vi "init.vi"(6 "Space size":i32=100000, 7 "Cleaneup":bool, 8 "error in (no error)":errorcluster) -> (0 "error out":errorcluster)   [LabVIEW 2015]
doc: "Initialize the tuple space naming it Spacename and reserving Space size locations for tuple. \nIf Cleanup is set to TRUE the pace will be initialized even if containing data.\nUse Cleneup=TRUE Spacesize=0 to deallocate all memory."
uses:
  LI_states.ctl
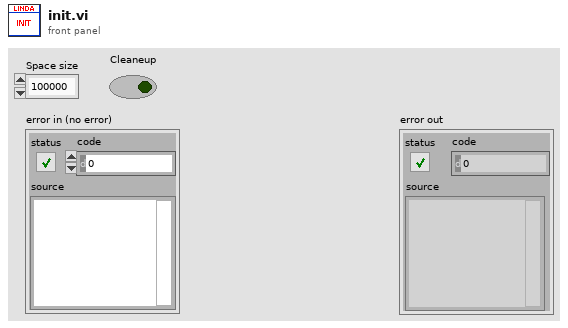
[diagram p1: front panel]
types:
  T1 = typedef "LI_states.ctl" = enum16{"Out", "In", "Rd", "Inp", "Rdp", "Init", "Cleanup", "RdAll"}
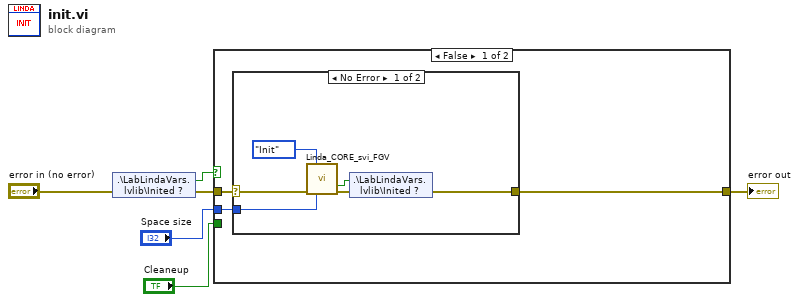
[diagram p0: block diagram]
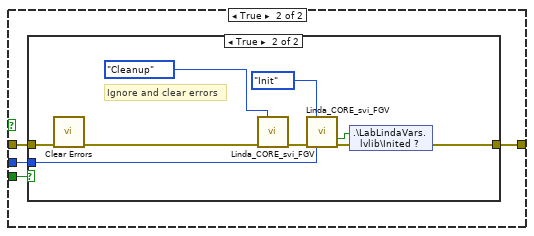
[diagram p3: hidden frame]
diagram:
  n1 = shared-variable ".\\LabLindaVars.lvlib\\Inited ?"(error in="error in (no error)") -> (w6:bool, error out=w4:errorcluster)
  n2 = case shown="False" w6 {
    tunnel: w4 -> [w7 w20]
    tunnel: [w9 w19] -> w3
    tunnel: "Cleaneup" -> [_ w18]
    tunnel: "Space size" -> [w8 w17]
    frame False {
      n3 = case shown="No Error" w7 {
        selector: w7 -> [w11 w16]
        tunnel: [w10 w16] -> w9
        tunnel: w8 -> [w12 _]
        frame No Error {
          n4 = call "Linda_CORE_svi_FGV.vi"("OP"=LI_states."Init", "error in (no error)"=w11, "Space size"=w12) -> ("Valid Op"=w13:bool, "error out"=w14:errorcluster)  [unwired: 8 in, 3 out]
          n5 = shared-variable ".\\LabLindaVars.lvlib\\Inited ?"(w13, error in=w14) -> (error out=w10:errorcluster)
        }
        frame Error {
        }
      }
    }
    frame True {
      n6 = case shown="True" w18 {
        tunnel: w20 -> [w21 w24]
        tunnel: [w21 w22] -> w19
        tunnel: w17 -> [_ w26]
        frame False {
        }
        frame True {
          # "Ignore and clear errors"
          n7 = call <vilib>:"Clear Errors.vi"("error in (no error)"=w24) -> ("error out"=w23:errorcluster)  [unwired: 5 in, 1 out]
          n8 = call "Linda_CORE_svi_FGV.vi"("OP"=LI_states."Cleanup", "error in (no error)"=w23) -> ("error out"=w25:errorcluster)  [unwired: 9 in, 4 out]
          n9 = call "Linda_CORE_svi_FGV.vi"("OP"=LI_states."Init", "error in (no error)"=w25, "Space size"=w26) -> ("Valid Op"=w27:bool, "error out"=w28:errorcluster)  [unwired: 8 in, 3 out]
          n10 = shared-variable ".\\LabLindaVars.lvlib\\Inited ?"(w27, error in=w28) -> (error out=w22:errorcluster)
        }
      }
    }
  }
  "error out" <- w3
